vi "copy - Vector Copy.vi"   [LabVIEW 2024, in "NI_AALBLAS.lvlib"]
doc: "<p>Replaces elements in <strong>y</strong> with elements in <strong>x</strong>.</p>"
uses:
  NI_AALBLAS.lvlib
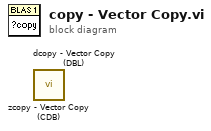
[diagram p0: block diagram]
diagram:
  n1 = call "zcopy - Vector Copy (CDB).vi"() -> ()  [unwired: 10 in, 2 out]
  n2 = call "dcopy - Vector Copy (DBL).vi"() -> ()  [unwired: 10 in, 2 out]
